vi "Update Transfer.vi"(8 "error in (no error)":errorcluster, 9 "data":string, 10 "Transfer":refnum<class "Transfer.lvclass">, 11 "UDP Transceiver in":refnum<class "UDP Transceiver.lvclass">) -> (0 "error out":errorcluster, 3 "UDP Transceiver out":refnum<class "UDP Transceiver.lvclass">)   [LabVIEW 2017, in "UDP.lvlib" / "UDP Transceiver.lvclass"]
uses:
  UDP Transceiver.lvclass
  Builds/Data Sharing Framework/Current/Core/DSF Core.lvlibp/Engine/Classes/Transfer/Transfer.lvclass
  UDP Size Mismatch Error.vi
  Builds/Data Sharing Framework/Current/Core/DSF Core.lvlibp/Engine/Classes/Buffer/Write Buffer 1D U8.vi
  Builds/Data Sharing Framework/Current/Core/DSF Core.lvlibp/Engine/Classes/Buffer/Buffer.lvclass
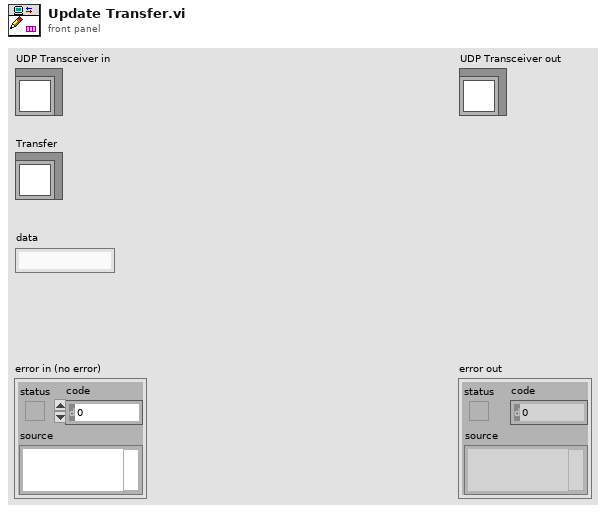
[diagram p1: front panel]
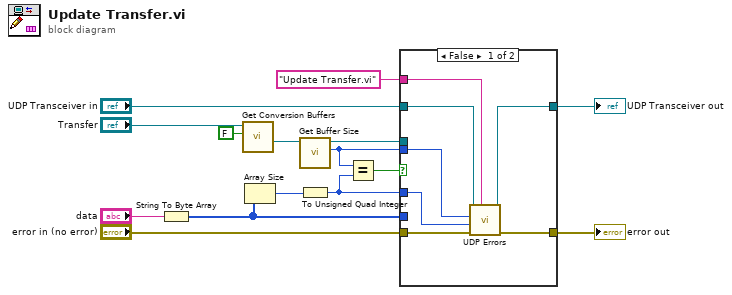
[diagram p0: block diagram]
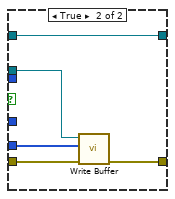
[diagram p2: hidden frame]
diagram:
  n1 = String To Byte Array(string="data") -> (unsigned byte array=w13:u8[])
  n2 = call "Get Conversion Buffers.vi"("inline?"=FALSE, "Transfer in"="Transfer") -> ("converted Buffer"=w3:refnum<class "Buffer.lvclass">)  [unwired: 6 in, 3 out]
  n3 = Array Size(array=w13) -> (size(s)=w15:i32)
  n4 = call "Get Buffer Size.vi"("Buffer in"=w3) -> ("buffer size"=w11:u64, "Buffer out"=w14:refnum<class "Buffer.lvclass">)  [unwired: 9 in]
  n5 = To Unsigned Quad Integer(1:w15) -> (0:w10:u64)
  n6 = Equal?(x=w11, y=w10) -> (x = y?=w12:bool)
  n7 = case shown="False" w12 {
    tunnel: w14 -> [_ w27]
    tunnel: "error in (no error)" -> [w22 w26]
    tunnel: [w21 w25] -> w6
    tunnel: w13 -> [_ w23]
    tunnel: "UDP Transceiver in" -> [w20 w24]
    tunnel: [w19 w24] -> w5
    tunnel: w11 -> [w17 _]
    tunnel: w10 -> [w18 _]
    tunnel: "Update Transfer.vi" ("source vi name") -> [w16 _]
    frame False {
      n8 = call-poly "UDP Errors.vi"("source vi name"=w16, "error in (no error)"=w22, "actual size"=w18, "expected size"=w17, "UDP in"=w20) -> ("error out"=w21:errorcluster, "UDP out"=w19:refnum<class "UDP Transceiver.lvclass">)  [unwired: 5 in]
    }
    frame True {
      n9 = call-poly "Write Buffer.vi"("error in (no error)"=w26, "src array in"=w23, "Buffer in"=w27) -> ("error out"=w25:errorcluster)  [unwired: 5 in, 3 out]
    }
  }
  "error out" <- w6
  "UDP Transceiver out" <- w5
